vi "SUB-BLE Rx data (Set)-Classify.vi"() -> (0 "data out":u8[](array[numeric]) format="%2x", 2 "Rx-data":bool=TRUE)   [LabVIEW 2015]
doc: "Use this template to create an application that executes repeatedly until you click the Stop button. This template polls the state of the Stop button and does not use events. Use the Top-Level Application template (not available in the Base package) to create a single-loop application with event handling."
uses:
  Global 1.vi
panel:
  out "BLE Packet (buf)":u8[](array[numeric])
  out "BLE Packet (data)":u8[](array[numeric])
  out "BLE Packet":bool=TRUE
  # "BLE 수신 데이터를 분류:  Setting Protocol"
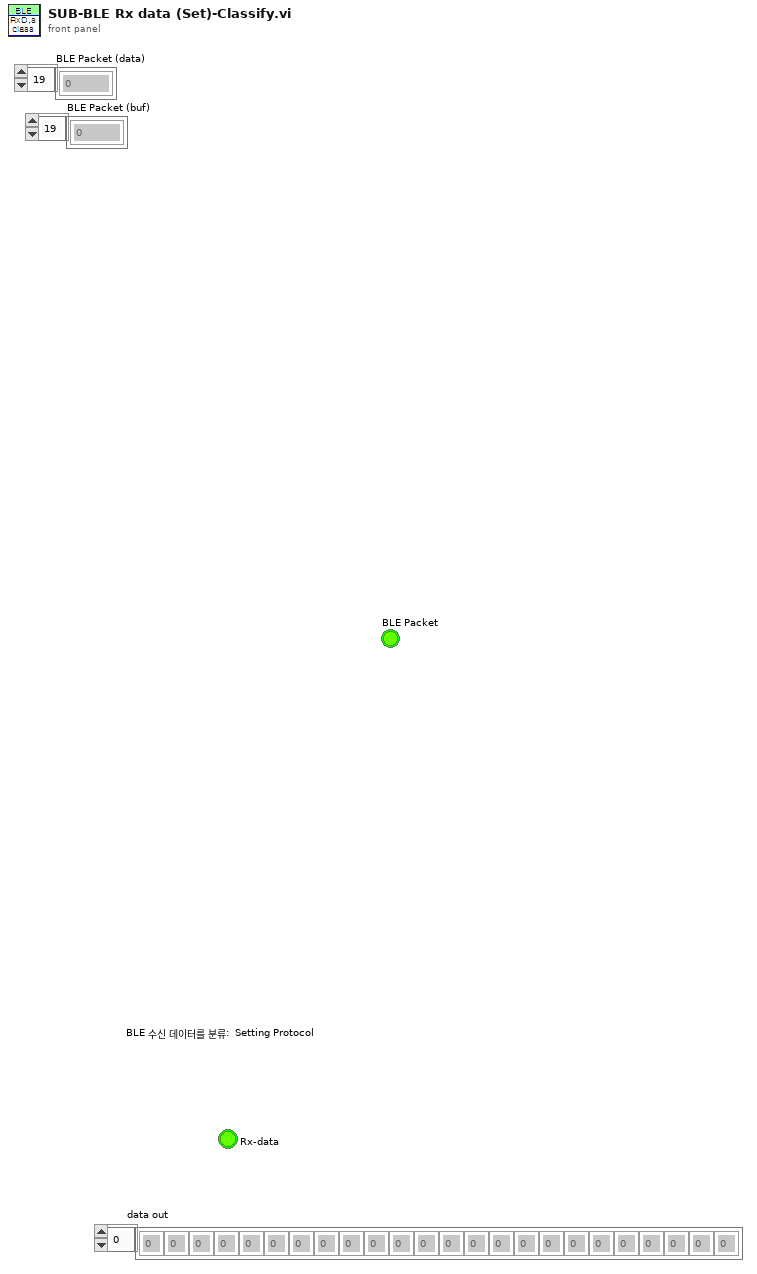
[diagram p1: front panel]
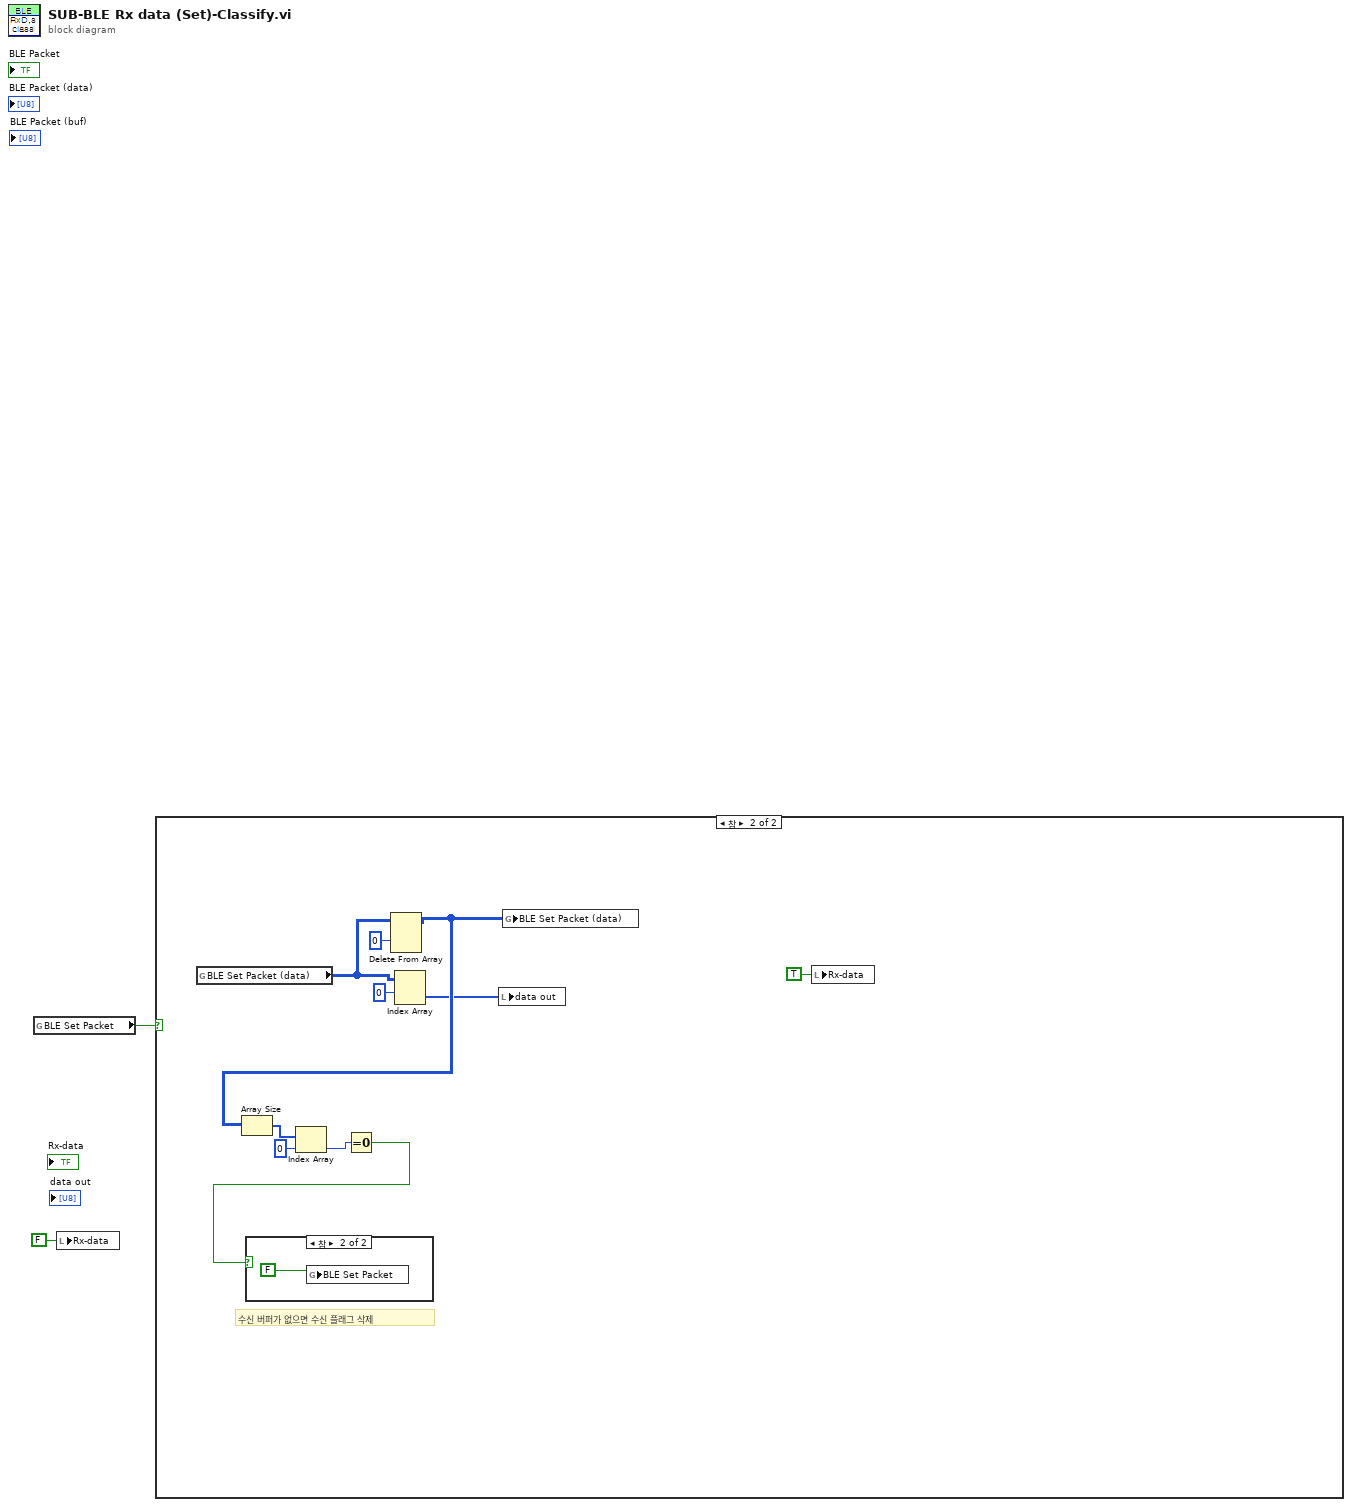
[diagram p0: block diagram]
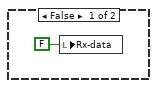
[diagram p2: hidden frame]
diagram:
  n1 = global read "Global 1.vi" "BLE Set Packet"() -> (w2:bool)
  n2 = local write "Rx-data"(FALSE ("Rx-mon")) -> ()
  n3 = case shown="참" w2 {
    frame False {
      n4 = local write "Rx-data"(FALSE ("Rx-mon")) -> ()
    }
    frame True {
      # "수신 버퍼가 없으면 수신 플래그 삭제"
      n5 = global read "Global 1.vi" "BLE Set Packet (data)"() -> (w12:u8[][])
      n6 = Delete From Array(array=w12, index (row)=0 ("인덱스 (행)")) -> (array with subset deleted=w10:u8[][])  [unwired: 2 in, 1 out]
      n7 = Array Size(array=w10) -> (size(s)=w9:i32[])
      n8 = Index Array(array=w9, index=0 ("인덱스")) -> (element=w7:i32)
      n9 = Equal To 0?(x=w7) -> (x = 0?=w6:bool)
      n10 = case shown="참" w6 {
        frame False {
        }
        frame True {
          n11 = global write "Global 1.vi" "BLE Set Packet"(FALSE ("BLE Packet")) -> ()
        }
      }
      n12 = Index Array(array=w12, index (row)=0 ("인덱스 (행)")) -> (element=w4:u8[])  [unwired: 1 in]
      n13 = local write "data out"(w4) -> ()
      n14 = global write "Global 1.vi" "BLE Set Packet (data)"(w10) -> ()
      n15 = local write "Rx-data"(TRUE ("Rx-mon")) -> ()
    }
  }
